vi "test.vi"() -> ()   [LabVIEW 2012]
panel:
  in  "Boolean 2":bool
  in  "Boolean":bool
  out "XY Graph":cluster{"Y":dbl[], "Y":dbl[]}[](graph)
  in  "Stop Button":bool
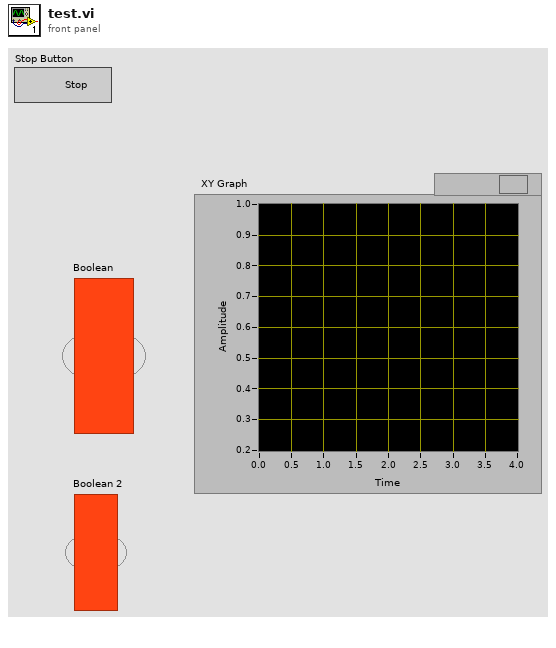
[diagram p1: front panel]
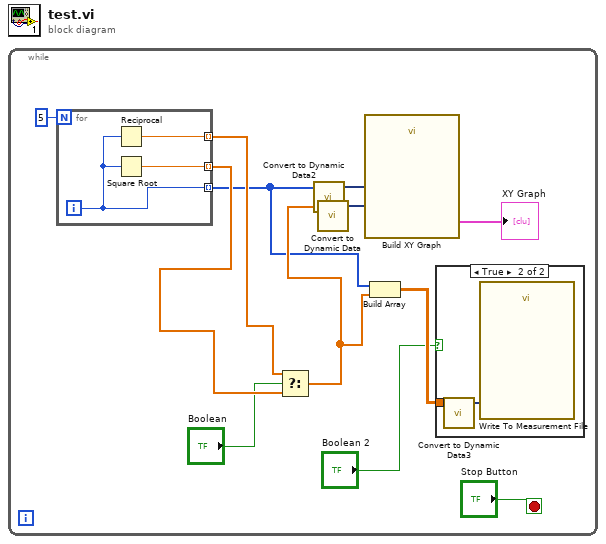
[diagram p0: block diagram]
diagram:
  n1 = while {
    stop <- "Stop Button" stop-if-true
    n2 = for {
      N: 5 -> [_]
      tunnel: [w15] -> w7 mode=indexing
      tunnel: [w17] -> w3 mode=indexing
      tunnel: [w16] -> w8 mode=indexing
      i -> [w17]
      n3 = Reciprocal(x=w17) -> (1/x=w16:dbl)
      n4 = Square Root(x=w17) -> (sqrt(x)=w15:dbl)
    }
    n5 = Select(t=w8, s="Boolean", f=w7) -> (s? t:f=w4:dbl[])
    n6 = call "Convert to Dynamic Data2"("Array"=w3) -> ("Dynamic Data Type"=w9:dynamicdata)  [unwired: 3 in]
    n7 = call "Convert to Dynamic Data"("Array"=w4) -> ("Dynamic Data Type"=w10:dynamicdata)  [unwired: 3 in]
    n8 = call "Build XY Graph"("Y Input"=w10, "X Input"=w9) -> ("XY Graph"=→"XY Graph":cluster{"Y":dbl[], "Y":dbl[]}[])  [unwired: 3 in, 6 out]
    n9 = Build Array(w3, w4) -> (w2:dbl[][])
    n10 = case shown="True" "Boolean 2" {
      tunnel: w2 -> [_ w14]
      frame False {
      }
      frame True {
        n11 = call "Convert to Dynamic Data3"("2D Array"=w14) -> ("Dynamic Data Type"=w13:dynamicdata)  [unwired: 3 in]
        n12 = call "Write To Measurement File"("Signals"=w13) -> ()  [unwired: 16 in, 3 out]
      }
    }
  }
